vi "IIR Filtering and Response.vi"() -> ()   [LabVIEW 2020]
doc: "Filters an input signal using the Infinite Impulse Response (IIR) filter design technique. You can specify the type of filter, such as low pass or band pass; filter topology, such as Butterworth or Chebyshev; and filter specifications, such as filter order or cutoff frequency. You can feed a single channel or multiple channels to the Digital IIR Filter VI used in this example."
uses:
  <vilib>/measure/macond.llb/Digital IIR Filter.vi
  <vilib>/measure/NI_MABase.lvlib
  <vilib>/measure/NI_MAPro.lvlib
panel:
  in  "display":T1(tab)
  out "Waveform Graph":waveform(dbl)[](graph)
  out "Magnitude response":cluster{"f0":dbl, "df":dbl, "Mag H(w)":dbl[]}(graph)={"f0"=0.0, "df"=0.9765625, "Mag H(w)"=[]}
  out "Phase response":cluster{"f0":dbl, "df":dbl, "Phase H(w)":dbl[]}(graph)={"f0"=0.0, "df"=0.9765625, "Phase H(w)"=[]}
  in  "specifications":T2(tab)
  in  "signal parameters":T3={"signal type"=enum."Sine Wave", "frequency"=101.0} {"frequency" format="%#.6g"}
  in  "sampling info":cluster{"Fs":dbl, "#s":dbl}={"Fs"=1000.0, "#s"=100.0} {"#s" step=100.0 format="%#.6g"; "Fs" step=1000.0 format="%0.2p"}
  in  "IIR filter specifications":T4={"Topology"=enum."Inverse Chebyshev", "Type"=enum."Lowpass", "Order"=10, "Lower Fc"=100.0, "Upper Fc"=200.0, "PB Ripple"=1.0, "SB Attenuation"=60.0} {"SB Attenuation" format="%#.6g"; "PB Ripple" format="%#.6g"; "Upper Fc" format="%#.6g"; "Lower Fc" format="%#.6g"}
  in  "reset signal":bool
  in  "reset filter":bool
  in  "N-waveforms 1-filter":T5(array[cluster])=[{"reset signal"=FALSE, "signal parameters"={"signal type"=enum."Sine Wave", "frequency"=101.0}, "sampling info"={"Fs"=1000.0, "#s"=100.0}}, {"reset signal"=FALSE, "signal parameters"={"signal type"=enum."Sine Wave", "frequency"=101.0}, "sampling info"={"Fs"=1000.0, "#s"=100.0}}] {"sampling info"."#s" step=100.0 format="%#.6g"; "sampling info"."Fs" step=1000.0 format="%0.2p"; "signal parameters"."frequency" format="%#.6g"}
  in  "IIR filter specifications (N)":T4={"Topology"=enum."Inverse Chebyshev", "Type"=enum."Lowpass", "Order"=10, "Lower Fc"=100.0, "Upper Fc"=200.0, "PB Ripple"=1.0, "SB Attenuation"=60.0} {"SB Attenuation" format="%#.6g"; "PB Ripple" format="%#.6g"; "Upper Fc" format="%#.6g"; "Lower Fc" format="%#.6g"}
  in  "reset filter":bool
  in  "N-waveforms N-filters":T6(array[cluster])=[{"IIR filter specifications"={"Topology"=enum."Inverse Chebyshev", "Type"=enum."Lowpass", "Order"=10, "Lower Fc"=100.0, "Upper Fc"=200.0, "PB Ripple"=1.0, "SB Attenuation"=60.0}, "reset signal"=FALSE, "signal parameters"={"signal type"=enum."Square Wave", "frequency"=100.0}, "sampling info"={"Fs"=1000.0, "#s"=100.0}}, {"IIR filter specifications"={"Topology"=enum."Inverse Chebyshev", "Type"=enum."Lowpass", "Order"=10, "Lower Fc"=100.0, "Upper Fc"=200.0, "PB Ripple"=1.0, "SB Attenuation"=60.0}, "reset signal"=FALSE, "signal parameters"={"signal type"=enum."Triangle Wave", "frequency"=100.0}, "sampling info"={"Fs"=10000.0, "#s"=1000.0}}] {"IIR filter specifications"."SB Attenuation" format="%#.6g"; "IIR filter specifications"."PB Ripple" format="%#.6g"; "IIR filter specifications"."Upper Fc" format="%#.6g"; "IIR filter specifications"."Lower Fc" format="%#.6g"; "sampling info"."#s" step=100.0 format="%#.6g"; "sampling info"."Fs" step=1000.0 format="%0.2p"; "signal parameters"."frequency" format="%#.6g"}
  in  "reset filters":bool
  in  "Stop":bool
  # "Overview: This example demonstrates the different polymorphic instances of the Digital IIR Filter VI.\nRequirements: LabVIEW Full Development System\nInstructions:\n1. Run the VI.\n2. Select different tabs.\n3. Interact with the filter specifications and signal parameters.\n4. Click Stop to stop the VI."
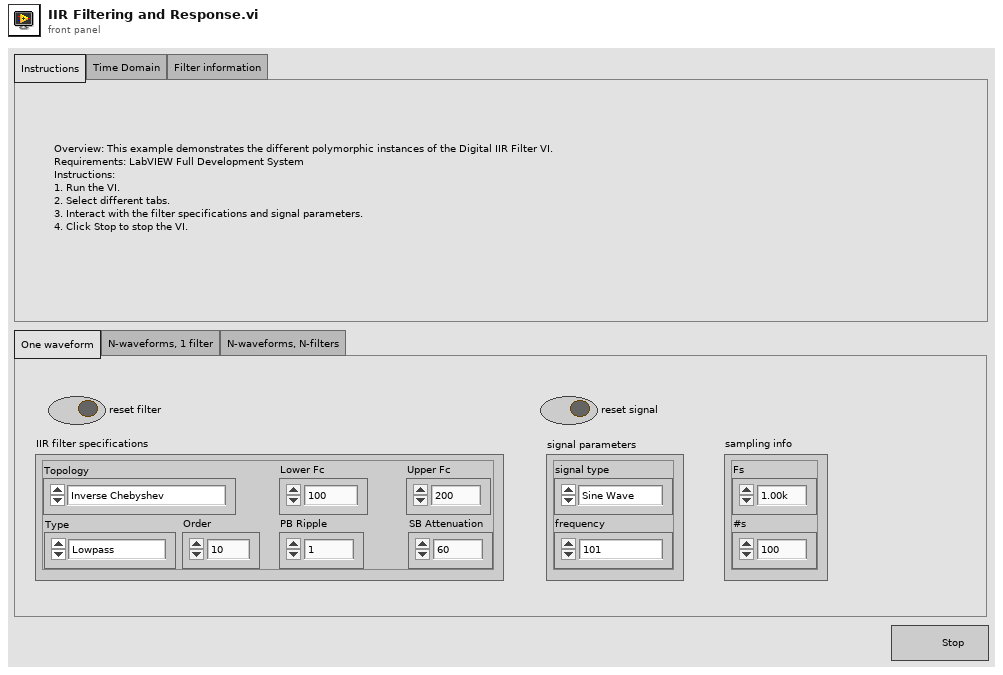
[diagram p1: front panel]
types:
  T1 = enum32{"Instructions", "Time Domain", "Filter information"}
  T2 = enum32{"One waveform", "N-waveforms, 1 filter", "N-waveforms, N-filters"}
  T3 = cluster{"signal type":enum16{"Sine Wave", "Triangle Wave", "Square Wave", "Sawtooth Wave"}, "frequency":dbl}
  T4 = cluster{"Topology":enum16{"Off", "Butterworth", "Chebyshev", "Inverse Chebyshev", "Elliptic", "Bessel"}, "Type":enum16{"Lowpass", "Highpass", "Bandpass", "Bandstop"}, "Order":i32, "Lower Fc":dbl, "Upper Fc":dbl, "PB Ripple":dbl, "SB Attenuation":dbl}
  T5 = cluster{"reset signal":bool, "signal parameters":cluster{"signal type":enum16{"Sine Wave", "Triangle Wave", "Square Wave", "Sawtooth Wave"}, "frequency":dbl}, "sampling info":cluster{"Fs":dbl, "#s":dbl}}[]
  T6 = cluster{"IIR filter specifications":cluster{"Topology":enum16{"Off", "Butterworth", "Chebyshev", "Inverse Chebyshev", "Elliptic", "Bessel"}, "Type":enum16{"Lowpass", "Highpass", "Bandpass", "Bandstop"}, "Order":i32, "Lower Fc":dbl, "Upper Fc":dbl, "PB Ripple":dbl, "SB Attenuation":dbl}, "reset signal":bool, "signal parameters":cluster{"signal type":enum16{"Sine Wave", "Triangle Wave", "Square Wave", "Sawtooth Wave"}, "frequency":dbl}, "sampling info":cluster{"Fs":dbl, "#s":dbl}}[]
  T7 = cluster{"magnitude H(w)":cluster{"f0":dbl, "df":dbl, "Mag H(w)":dbl[]}, "phase H(w)":cluster{"f0":dbl, "df":dbl, "Phase H(w)":dbl[]}, "order":i32}[]
  T8 = cluster{"magnitude H(w)":cluster{"f0":dbl, "df":dbl, "Mag H(w)":dbl[]}, "phase H(w)":cluster{"f0":dbl, "df":dbl, "Phase H(w)":dbl[]}, "order":i32}
  T9 = enum16{"Sine Wave", "Triangle Wave", "Square Wave", "Sawtooth Wave"}
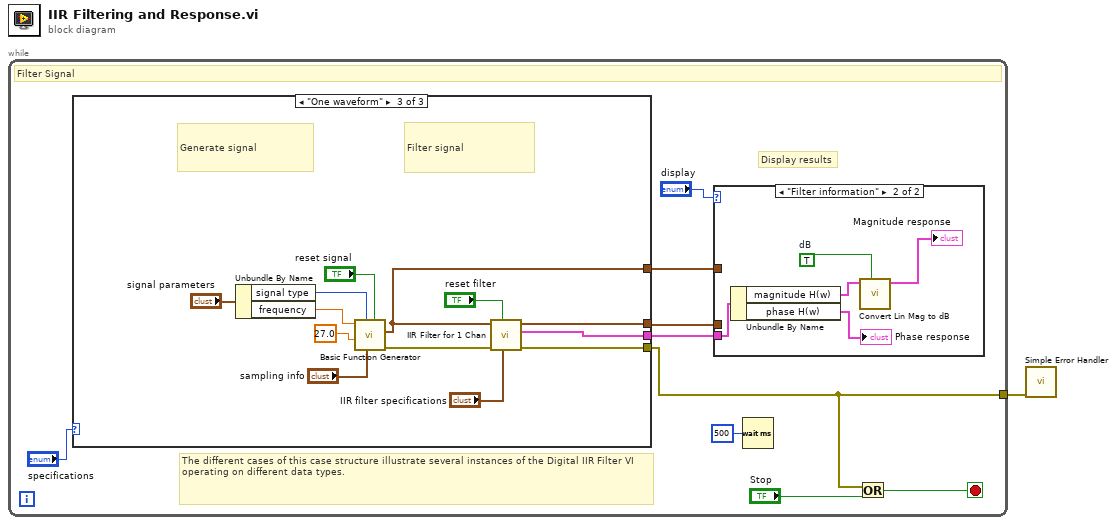
[diagram p0: block diagram]
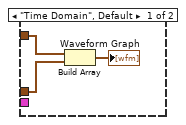
[diagram p2: hidden frame]
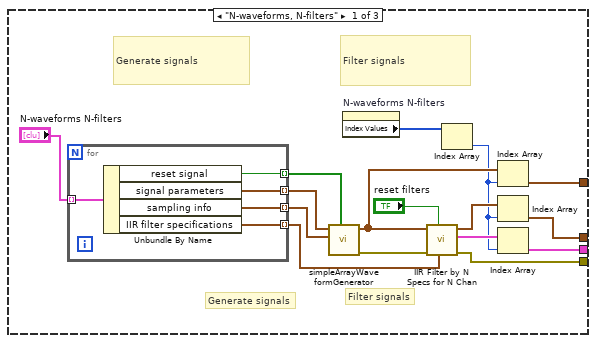
[diagram p3: hidden frame]
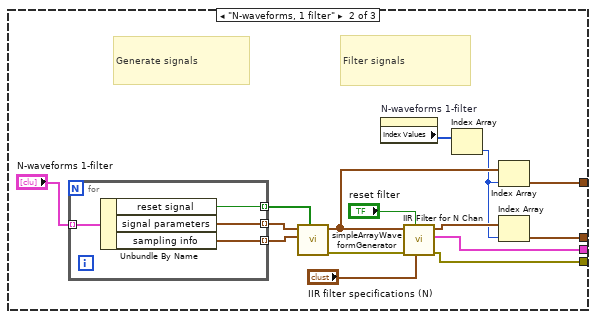
[diagram p4: hidden frame]
diagram:
  n1 = while {
    tunnel: [w2] -> w1
    stop <- w9 stop-if-true
    # "The different cases of this case structure illustrate several instances of the Digital IIR Filter VI operating on different data types."
    # "Display results"
    # "Filter Signal"
    n2 = case shown="\"One waveform\"" "specifications" {
      tunnel: [w34 w40 w71] -> w2
      tunnel: [w33 w54 w68] -> w6
      tunnel: [w32 w53 w67] -> w5
      tunnel: [w29 w51 w69] -> w7
      frame "N-waveforms, N-filters" {
        # "Filter signals"
        # "Generate signals"
        # "Filter signals"
        # "Generate signals"
        n3 = for {
          tunnel: "N-waveforms N-filters" -> [w39] mode=indexing
          tunnel: [w38] -> w25 mode=indexing
          tunnel: [w37] -> w24 mode=indexing
          tunnel: [w36] -> w23 mode=indexing
          tunnel: [w35] -> w22 mode=indexing
          n4 = Unbundle By Name(w39) -> ("reset signal"=w38:bool, "signal parameters"=w37:T3, "sampling info"=w36:cluster{"Fs":dbl, "#s":dbl}, "IIR filter specifications"=w35:T4)
        }
        n5 = call "simpleArrayWaveformGenerator.vi"("reset signal"=w25, "sampling info"=w23, "signal parameters"=w24) -> ("error out"=w27:errorcluster, "signal(s) in"=w28:waveform(dbl)[])  [unwired: 7 in]
        n6 = property on="N-waveforms N-filters" class="Arr (strict)"() -> ("Index Values"=w21:u32[])  [unwired: 2 in, 2 out]
        n7 = call-poly <vilib>:"IIR Filter by N Specs for N Chan.vi"("IIR filter specifications"=w22, "reset filters"="reset filters", "error in (no error)"=w27, "signal(s) in"=w28) -> ("error out"=w34:errorcluster, "filter information"=w30:T7, "signal(s) out"=w31:waveform(dbl)[])  [unwired: 5 in]
        n8 = Index Array(array=w21) -> (element=w20:u32)  [unwired: 1 in]
        n9 = Index Array(array=w28, index=w20) -> (element=w33:waveform(dbl))
        n10 = Index Array(array=w31, index=w20) -> (element=w32:waveform(dbl))
        n11 = Index Array(array=w30, index=w20) -> (element=w29:T8)
      }
      frame "N-waveforms, 1 filter" {
        # "Filter signals"
        # "Generate signals"
        n12 = for {
          tunnel: "N-waveforms 1-filter" -> [w58] mode=indexing
          tunnel: [w57] -> w47 mode=indexing
          tunnel: [w56] -> w46 mode=indexing
          tunnel: [w55] -> w45 mode=indexing
          n13 = Unbundle By Name(w58) -> ("reset signal"=w57:bool, "signal parameters"=w56:T3, "sampling info"=w55:cluster{"Fs":dbl, "#s":dbl})
        }
        n14 = call "simpleArrayWaveformGenerator.vi"("reset signal"=w47, "sampling info"=w45, "signal parameters"=w46) -> ("error out"=w50:errorcluster, "signal(s) in"=w49:waveform(dbl)[])  [unwired: 7 in]
        n15 = property on="N-waveforms 1-filter" class="Arr (strict)"() -> ("Index Values"=w44:u32[])  [unwired: 2 in, 2 out]
        n16 = call-poly <vilib>:"IIR Filter for N Chan.vi"("IIR filter specifications"="IIR filter specifications (N)", "reset filters"="reset filter", "error in (no error)"=w50, "signal(s) in"=w49) -> ("error out"=w40:errorcluster, "filter information"=w51:T8, "signal(s) out"=w52:waveform(dbl)[])  [unwired: 5 in]
        n17 = Index Array(array=w44) -> (element=w43:u32)  [unwired: 1 in]
        n18 = Index Array(array=w49, index=w43) -> (element=w54:waveform(dbl))
        n19 = Index Array(array=w52, index=w43) -> (element=w53:waveform(dbl))
      }
      frame "One waveform" {
        # "Filter signal"
        # "Generate signal"
        n20 = Unbundle By Name("signal parameters") -> ("signal type"=w66:T9, "frequency"=w65:dbl)
        n21 = call <vilib>:"Basic Function Generator.vi"("reset signal"="reset signal", "sampling info"="sampling info", "signal type"=w66, "phase"=27.0, "frequency"=w65) -> ("error out"=w70:errorcluster, "signal out"=w68:waveform(dbl))  [unwired: 4 in, 1 out]
        n22 = call-poly <vilib>:"IIR Filter for 1 Chan.vi"("IIR filter specifications"="IIR filter specifications", "reset filter"="reset filter", "error in (no error)"=w70, "signal in"=w68) -> ("error out"=w71:errorcluster, "filter information"=w69:T8, "signal out"=w67:waveform(dbl))  [unwired: 5 in]
      }
    }
    n23 = case shown="\"Filter information\"" "display" {
      tunnel: w7 -> [_ w18]
      tunnel: w6 -> [w13 _]
      tunnel: w5 -> [w12 _]
      frame "Time Domain", Default {
        n24 = Build Array(w13, w12) -> (→"Waveform Graph":waveform(dbl)[])
      }
      frame "Filter information" {
        w16 = TRUE  # dB
        n25 = Unbundle By Name(w18) -> ("magnitude H(w)"=w17:cluster{"f0":dbl, "df":dbl, "Mag H(w)":dbl[]}, "phase H(w)"=→"Phase response":cluster{"f0":dbl, "df":dbl, "Phase H(w)":dbl[]})
        n26 = call "Convert Lin Mag to dB.vi"("convert to dB"=w16, "magnitude H(w)"=w17) -> ("magnitude H(w) in dB"=→"Magnitude response":cluster{"f0":dbl, "df":dbl, "Mag H(w)":dbl[]})  [unwired: 9 in]
      }
    }
    n27 = Wait (ms)(milliseconds to wait=u32 500) -> ()  [unwired: 1 out]
    n28 = Or(x=w2, y="Stop") -> (x .or. y?=w9:bool)
  }
  n29 = call <vilib>:"Simple Error Handler.vi"("error in (no error)"=w1) -> ()  [unwired: 4 in, 5 out]
